vi "ReadDeviceData.vi"(11 "Device Data in":T1 {"IDS" format="%.0x"; "IDL" format="%.0x"; "IDM" format="%.0x"; "IDH" format="%.0x"}) -> (0 "Error Out":errorcluster, 1 "Message":string, 2 "Device Data out":T1 {"IDS" format="%.0x"; "IDL" format="%.0x"; "IDM" format="%.0x"; "IDH" format="%.0x"}, 3 "Function Output Comment":string)   [LabVIEW 2019]
uses:
  Device Data.ctl
  164J027_AD/Brooks DLL 1.0.1.0 32bit/Brooks DLL 1.0.1.0 Release 10032016/S Protocol/BrooksDLL.dll
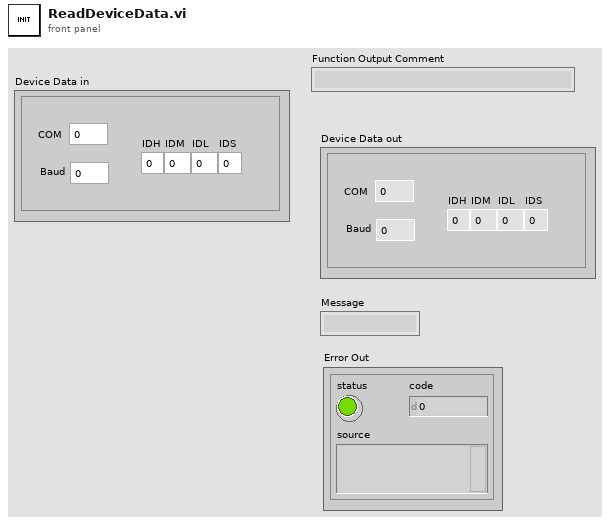
[diagram p1: front panel]
types:
  T1 = typedef "Device Data.ctl" = cluster{"COM":i32, "Baud":i32, "IDH":u8, "IDM":u8, "IDL":u8, "IDS":u8}
  T2 = cluster{bool, "return type":i32, "Function Output Comment":string}
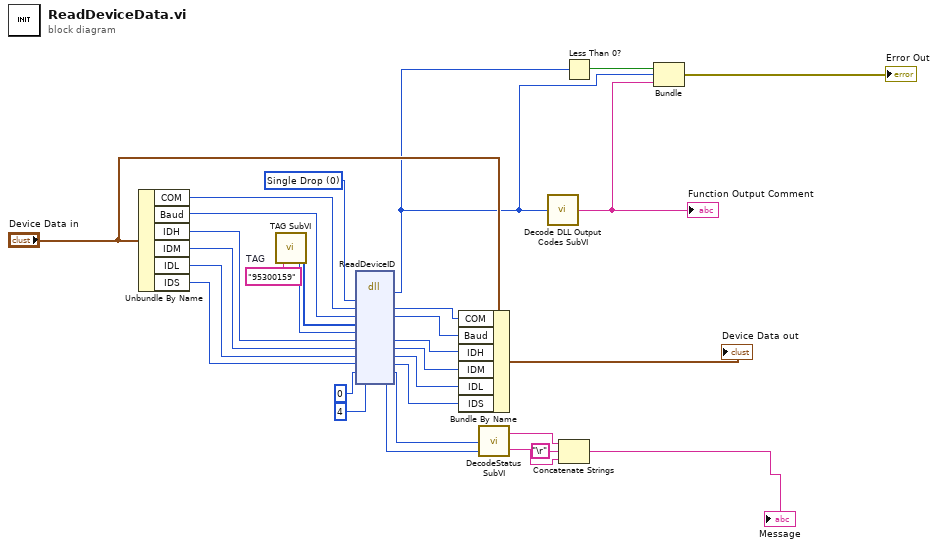
[diagram p0: block diagram]
diagram:
  w7 = "95300159"  # TAG
  w12 = 0 items=["Single Drop", "Multi-Drop"] ("Drop Type")
  n1 = Unbundle By Name("Device Data in") -> ("COM"=w19:i32, "Baud"=w20:i32, "IDH"=w21:u8, "IDM"=w22:u8, "IDL"=w23:u8, "IDS"=w24:u8)
  n2 = call "TAG SubVI.vi"("TAG String"=w7) -> ("TAG"=w10:u8[], "Length"=w11:i32)
  n3 = dll-call lib="G:/Developpement_de_Programmes/Programmes/Controle de pression/164J027_AD/Brooks DLL 1.0.1.0 32bit/Brooks DLL 1.0.1.0 Release 10032016/S Protocol/BrooksDLL.dll" fn="ReadDeviceID"("DropType"=w12, "COM"=w19, "Baud"=w20, "TAG"=w10, "Length"=w11, "IDH"=w21, "IDM"=w22, "IDL"=w23, "IDS"=w24, "S1"=u8 0, "S2"=u8 4) -> ("return type"=w3:i32, "COM"=w5:i32, "Baud"=w6:i32, "IDH"=w25:u8, "IDM"=w26:u8, "IDL"=w27:u8, "IDS"=w28:u8, "S1"=w9:u8, "S2"=w8:u8)  [unwired: 6 in, 2 out]
  n4 = Bundle By Name(cluster="Device Data in", "COM"=w5, "Baud"=w6, "IDH"=w25, "IDM"=w26, "IDL"=w27, "IDS"=w28) -> (→"Device Data out":T1)
  n5 = call "DecodeStatus SubVI.vi"("S2"=w8, "S1"=w9) -> ("S2 String"=w17:string, "S1 String"=w16:string)
  n6 = call "Decode DLL Output Codes SubVI.vi"("Numeric"=w3) -> ("Function Output Comment"=w2:string)
  "Function Output Comment" <- w2
  n7 = Concatenate Strings(w16, "\r" ("string"), w17) -> (→"Message":string)
  n8 = Less Than 0?(x=w3) -> (x < 0?=w4:bool)
  n9 = Bundle(w4, "return type"=w3, "Function Output Comment"=w2) -> (→"Error Out":T2)  [unwired: 1 in]
